vi "Logout.vi"(8 "error in (no error)":errorcluster, 11 "TestBench in":refnum<class "TestBench.lvclass">) -> (0 "error out":errorcluster, 3 "TestBench out":refnum<class "TestBench.lvclass">)   [LabVIEW 2019, in "TestBench.lvlib" / "TestBench.lvclass"]
uses:
  TestBench.lvclass
  TestBench.lvclass/TestBench.ctl
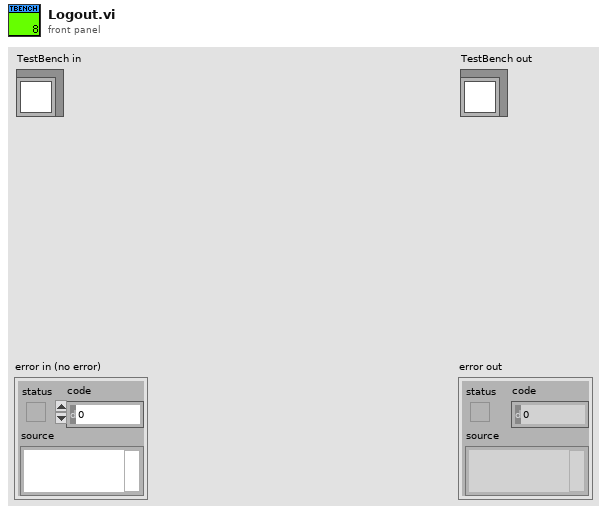
[diagram p1: front panel]
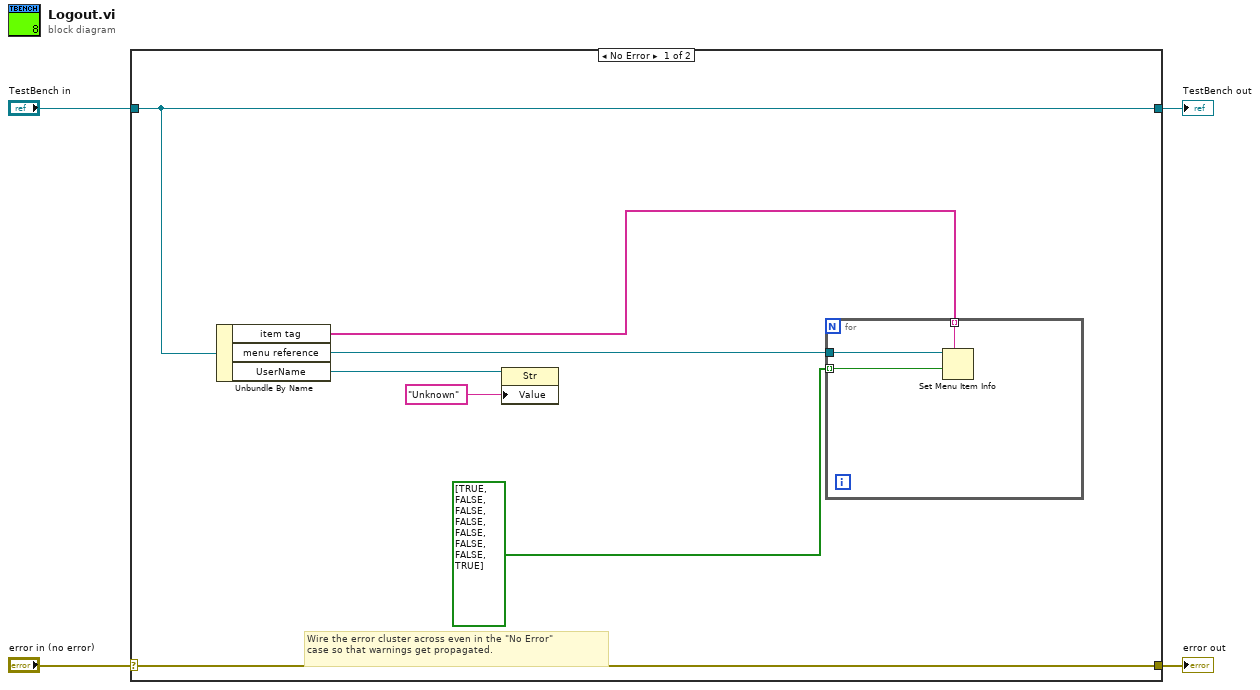
[diagram p0: block diagram]
diagram:
  n1 = case shown="No Error" "error in (no error)" {
    selector: "error in (no error)" -> [w11 w16]
    tunnel: [w11 w16] -> w3
    tunnel: [w6 w15] -> w1
    tunnel: "TestBench in" -> [w6 w15]
    frame No Error {
      # "Wire the error cluster across even in the \"No Error\"\ncase so that warnings get propagated."
      n2 = Unbundle By Name(w6) -> ("item tag"=w5:string[], "menu reference"=w9:refnum<k9>, "UserName"=w10:refnum<vi>)
      n3 = property class="Str"(reference=w10, "Value"="Unknown") -> ()  [unwired: 1 in, 2 out]
      n4 = for {
        tunnel: w9 -> [w14]
        tunnel: w5 -> [w13] mode=indexing
        tunnel: bool[] [TRUE, FALSE, FALSE, FALSE, FALSE, FALSE, FALSE, TRUE] -> [w12] mode=indexing
        n5 = Set Menu Item Info(7:w13, 9:w12, 11:w14) -> ()  [unwired: 4 in, 2 out]
      }
    }
    frame Error {
    }
  }
  "error out" <- w3
  "TestBench out" <- w1
